vi "robot wait stop.vi"(0 "robot_id":i32, 11 "error in (no error)":errorcluster caption="错误输入（无错误）") -> (4 "robot_id out":i32, 8 "function return":i32, 15 "error out":errorcluster caption="错误输出")   [LabVIEW 2020, in "small_scara_interface.lvlib"]
doc: "extern \"C\" __declspec(dllexport) int robot_wait_stop(int robot_id);"
uses:
  small_scara_interface.lvlib
  small_scara_interface.dll
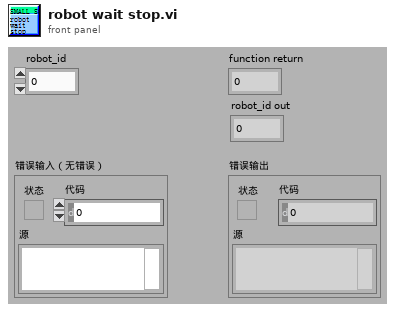
[diagram p1: front panel]
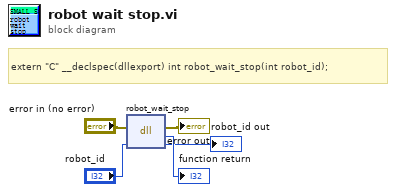
[diagram p0: block diagram]
diagram:
  # "extern \"C\" __declspec(dllexport) int robot_wait_stop(int robot_id);"
  n1 = dll-call lib="C:/Users/15239/Desktop/labview multichannel v314/subvi/robot/subvi/Robot-HL/small_scara_interface/small_scara_interface.*" fn="robot_wait_stop"(error in="error in (no error)", "robot_id"="robot_id") -> (error out=→"error out":errorcluster, "返回类型"=→"function return":i32, "robot_id"=→"robot_id out":i32)  [unwired: 2 in, 1 out]
